vi "Auton-Pickup.vi"(8 "error in (no error)":errorcluster, 10 "ToHeight":dbl, 11 "Auton Event Queue Data":refnum<queue>) -> (0 "error out":errorcluster, 2 "Done":bool, 3 "Auton Event Queue Data 2":refnum<queue>)   [LabVIEW 2014]
uses:
  Robot Global Data.vi
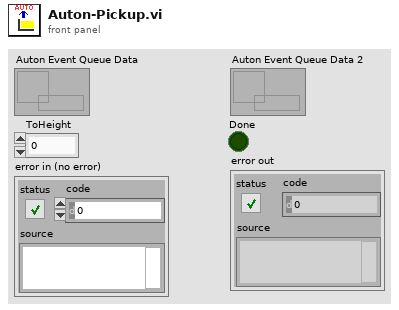
[diagram p1: front panel]
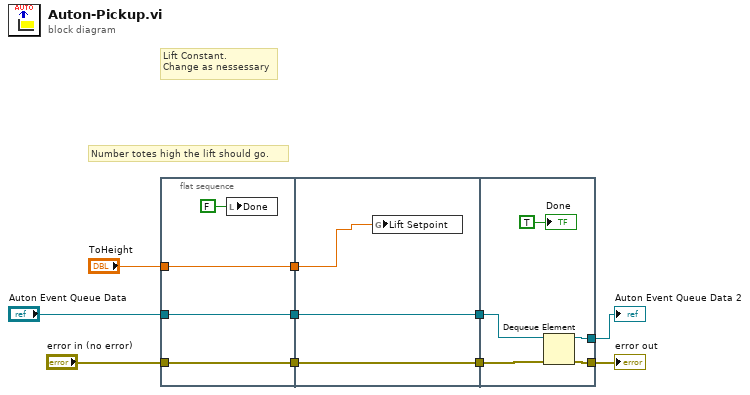
[diagram p0: block diagram]
diagram:
  # "Number totes high the lift should go."
  # "Lift Constant.\nChange as nessessary"
  n1 = flat-sequence {
    tunnel: "ToHeight" -> [w14]
    tunnel: [w14] -> w9
    tunnel: "Auton Event Queue Data" -> [w12]
    tunnel: [w12] -> w7
    tunnel: "error in (no error)" -> [w11]
    tunnel: [w11] -> w4
    tunnel: w9 -> [w15]
    tunnel: w7 -> [w17]
    tunnel: [w17] -> w6
    tunnel: w4 -> [w16]
    tunnel: [w16] -> w3
    tunnel: w6 -> [w20]
    tunnel: w3 -> [w21]
    tunnel: [w19] -> w2
    tunnel: [w18] -> w1
    frame #0 {
      n2 = local write "Done"(FALSE ("Done")) -> ()
    }
    frame #1 {
      n3 = global write "Robot Global Data.vi" "Lift Setpoint"(w15) -> ()
    }
    frame #2 {
      n4 = Dequeue Element(queue=w20, error in (no error)=w21) -> (queue out=w19:refnum<queue>, error out=w18:errorcluster)  [unwired: 1 in, 2 out]
      "Done" <- TRUE
    }
  }
  "error out" <- w1
  "Auton Event Queue Data 2" <- w2
